vi "RemotePanelMethods-Client_TerraNova.vi"() -> ()   [LabVIEW 2009]
doc: "This VI illustrates how to programmatically connect to a remote front panel. It utilizes the new VI server properties and methods introduced in LabVIEW 7.0. A connection is established to the specified VI and control can also be requested. Once control is requested, the VI can only be run once since the server will close the connection automatically after one run. This VI is used in conjunction with the Remote Panel Server.vi example."
panel:
  in  "Req Ctl":bool caption="Request Control"
  in  "Web Server Port":i32=80
  in  "Server Address":string="s132pc1.ssrl-beam.slac.stanford.edu"
  in  "VI Name":string="Terranova908A.vi"
  # "Instructions:  \n1.  Open the Remote Panel Server.vi example that is used in conjunction with this example and run it.\n     NOTE:This must be done in another LabVIEW of the same version since a remote panel connection\n     cannot be made from a LabVIEW to itself.\n2.  Specify the address and web server port of the server.\n     (If the VI name is changed, the server must also be configured for that VI.) \n3.  Run this VI and then click on \"Request Control\" to control the VI.\n4.  Run the Power Spectrum Example and when you are done stop the VI.\n5.  Note that you are disconnected from the server automatically since it is configured to only let you\n     run the VI once."
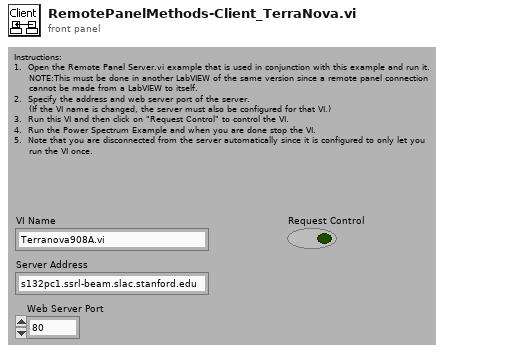
[diagram p1: front panel]
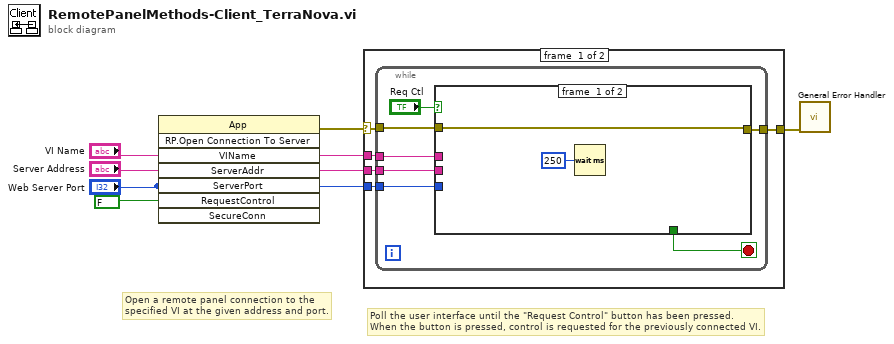
[diagram p0: block diagram]
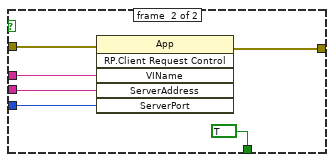
[diagram p2: hidden frame]
diagram:
  # "Poll the user interface until the \"Request Control\" button has been pressed.\nWhen the button is pressed, control is requested for the previously connected VI."
  # "Open a remote panel connection to the\nspecified VI at the given address and port."
  n1 = invoke class="App" method="RP.Open Connection To Server"("VIName"="VI Name", "ServerAddr"="Server Address", "ServerPort"="Web Server Port", "RequestControl"=FALSE) -> (error out=w2:errorcluster)  [unwired: 4 in, 7 out]
  n2 = case shown="No Error" w2 {
    selector: w2 -> [w7 w27]
    tunnel: "VI Name" -> [w11 _]
    tunnel: "Server Address" -> [w10 _]
    tunnel: "Web Server Port" -> [w9 _]
    tunnel: [w8 w27] -> w1
    frame #0 {
      n3 = while {
        tunnel: w11 -> [w16]
        tunnel: w10 -> [w15]
        tunnel: w9 -> [w14]
        tunnel: w7 -> [w13]
        tunnel: [w12] -> w8
        stop <- w18 stop-if-true
        n4 = case shown="True" "Req Ctl" {
          tunnel: [_ TRUE] -> w18
          tunnel: w16 -> [_ w25]
          tunnel: w15 -> [_ w24]
          tunnel: w14 -> [_ w23]
          tunnel: w13 -> [w19 w22]
          tunnel: [w19 w21] -> w12
          frame #0 {
            n5 = Wait (ms)(milliseconds to wait=u32 250) -> ()  [unwired: 1 out]
          }
          frame #1 {
            n6 = invoke class="App" method="RP.Client Request Control"(error in=w22, "VIName"=w25, "ServerAddress"=w24, "ServerPort"=w23) -> (error out=w21:errorcluster)  [unwired: 2 in, 5 out]
          }
        }
      }
    }
    frame #1 {
    }
  }
  n7 = call <vilib>:"General Error Handler.vi"("error in (no error)"=w1) -> ()  [unwired: 10 in, 5 out]
